vi "fpga_Counter.vi"(7 "reset":bool, 9 "Input Valid?":bool, 11 "upper limit":fxp<+,5,5>) -> (1 "Multichannel Valid?":bool, 3 "count":fxp<+,5,5>)   [LabVIEW 2011, in "NI_EP_Resample_FPGA.lvlib"]
uses:
  <vilib>/rvi/FXPMathLib/basic elements/FxpAddSub/XNode/nifxpmath_AddSub.xnode
  <vilib>/addons/Electrical Power/PQ/Resampling/NI_EP_Resample_FPGA.lvlib
  <vilib>/rvi/FXPMathLib/sim/FxpSim.dll
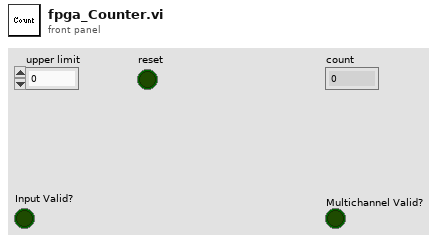
[diagram p1: front panel]
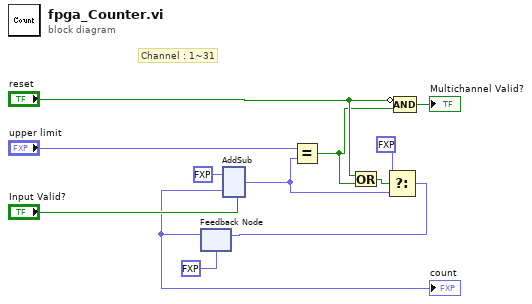
[diagram p0: block diagram]
diagram:
  # "Channel : 1~31"
  n1 = feedback #1(fxp<+,5,5> 0.0 ("s")) -> (w4:fxp<+,5,5>)
  "count" <- w4
  n2 = xnode "AddSub"("x"=fxp<+,5,5> 0.0 ("s"), "y"=w4, "carry-in"="Input Valid?") -> ("s"=w8:fxp<+,5,5>)  [unwired: 1 out]
  n3 = Equal?(x="upper limit", y=w8) -> (x = y?=w2:bool)
  n4 = Or(x="reset", y=w2) -> (x .or. y?=w1:bool)
  n5 = Select(t=fxp<+,5,5> 0.0 ("s"), s=w1, f=w8) -> (s? t:f=w6:fxp<+,5,5>)
  n6 = feedback-in #1(w6) -> ()
  n7 = Compound Arithmetic op=AND(invert "reset", w2) -> (→"Multichannel Valid?":bool)
